vi "CreatePrivateEvents.vi"(8 "error in (no error)":errorcluster, 11 "Tool Data":refnum<class "Tool Data.lvclass">) -> (0 "error out":errorcluster, 3 "Tool Data out":refnum<class "Tool Data.lvclass">)   [LabVIEW 2019, in "Tool Data.lvclass"]
doc: "---------------------------------------------------------------\nJKI State Machine Objects™\nhttp://jki.net/state-machine-objects/\nCopyright (C) 2005-2015, JKI <info@jki.net>\nALL RIGHTS RESERVEDJKI State Machine Objects (SMO) 1.0.0.4\nJKI - JKI\nCopyright (c) 2015, JKI"
uses:
  Tool Data.lvclass
  Typedefs/PrivateEvents--Tool Data.Update Objects.ctl
  Settings/Setting Database/Typedefs/PublicEvents--Setting Database.PathsUpdated.ctl
  Settings/Path Settings/Path Settings.lvclass
  Settings/Setting Database/Typedefs/PublicEvents--Setting Database.RectanglesUpdated.ctl
  Settings/Rectangle Settings/Rectangle Settings.lvclass
  Settings/Setting Database/Typedefs/PublicEvents--Setting Database.FunnelsUpdated.ctl
  Settings/Funnel Settings/Funnel Settings.lvclass
  Settings/Setting Database/Typedefs/PublicEvents--Setting Database.DotsUpdated.ctl
  Settings/Dot Settings/Dot Settings.lvclass
  Parse/ParsePaths/Path.lvclass
  Parse/Rectangle/Rectangle.lvclass
  Parse/Image/SVGImage.lvclass
  Parse/Dot/Dot.lvclass
  Tool Data.lvclass/Tool Data.ctl
  <vilib>/JKI/JKI SMO/SMO/SMO.lvclass
  Settings/Setting Database/Setting Database.lvclass
panel:
  # "For instructions on how to use the JKI State Machine Objects, examples and video tutorials, visit:\nhttp://jki.net/state-machine-objects/\n\nJKI State Machine Objects™\nhttp://jki.net/state-machine-objects/\nCopyright (C) 2005-2015, JKI <info@jki.net>\nALL RIGHTS RESERVED"
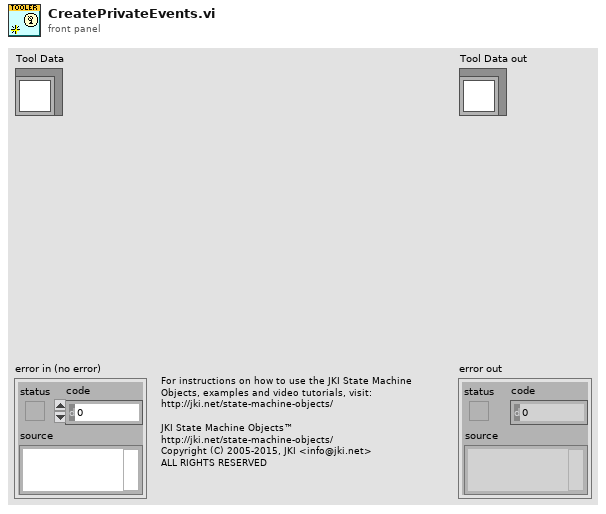
[diagram p1: front panel]
types:
  T1 = typedef "Tool Data.lvclass/PrivateEvents--Tool Data.Update Objects.ctl" = cluster{"Settings":cluster{"Paths":T2, "Rectangles":T3, "Funnels":T4, "Dots":T5}, "Data":cluster{"Paths":refnum<class "Path.lvclass">[], "Rectangles":refnum<class "Rectangle.lvclass">[], "SVGImage":refnum<class "SVGImage.lvclass">, "Dots":refnum<class "Dot.lvclass">[], "Funnels":refnum<class "Path.lvclass">[]}}
  T2 = typedef "Setting Database.lvclass/PublicEvents--Setting Database.PathsUpdated.ctl" = refnum<class "Path Settings.lvclass">[]
  T3 = typedef "Setting Database.lvclass/PublicEvents--Setting Database.RectanglesUpdated.ctl" = refnum<class "Rectangle Settings.lvclass">[]
  T4 = typedef "Setting Database.lvclass/PublicEvents--Setting Database.FunnelsUpdated.ctl" = refnum<class "Funnel Settings.lvclass">[]
  T5 = typedef "Setting Database.lvclass/PublicEvents--Setting Database.DotsUpdated.ctl" = refnum<class "Dot Settings.lvclass">[]
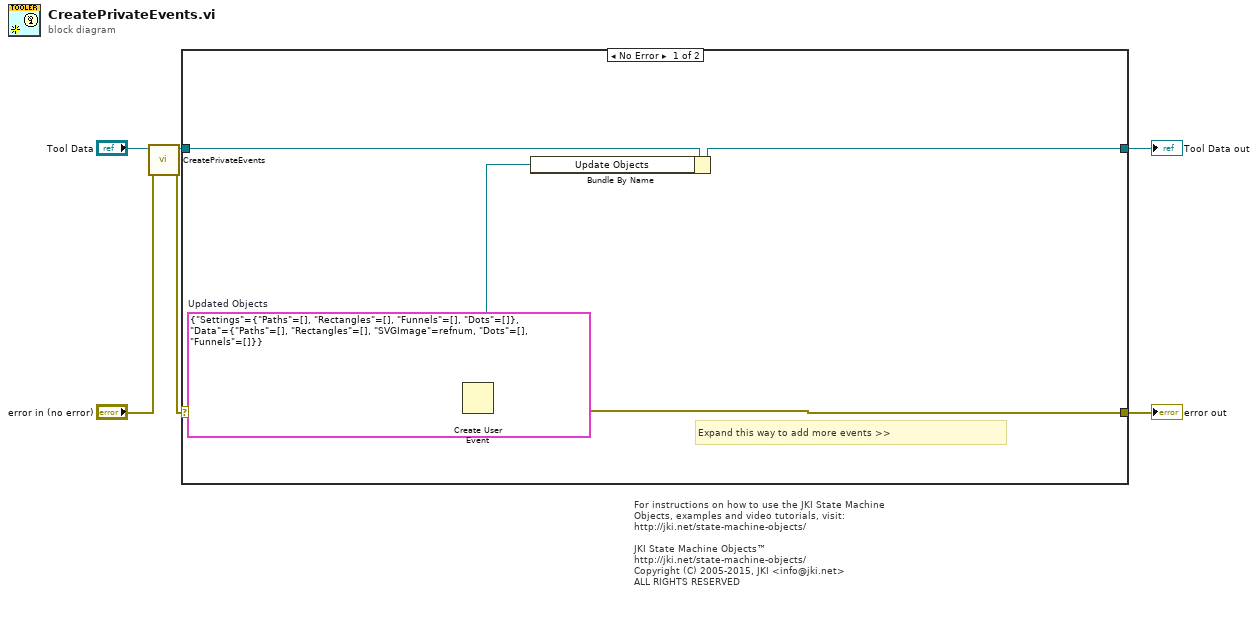
[diagram p0: block diagram]
diagram:
  # "For instructions on how to use the JKI State Machine Objects, examples and video tutorials, visit:\nhttp://jki.net/state-machine-objects/\n\nJKI State Machine Objects™\nhttp://jki.net/state-machine-objects/\nCopyright (C) 2005-2015, JKI <info@jki.net>\nALL RIGHTS RESERVED"
  n1 = call-parent "CreatePrivateEvents.vi"("error in (no error)"="error in (no error)", "SMO"="Tool Data") -> ("error out"=w1:errorcluster, "SMO out"=w3:refnum<class "Tool Data.lvclass">)  [unwired: 8 in]
  n2 = case shown="No Error" w1 {
    selector: w1 -> [w11 w14]
    tunnel: [w9 w14] -> w5
    tunnel: [w10 w13] -> w6
    tunnel: w3 -> [w12 w13]
    frame No Error {
      w8 = T1 {"Settings"={"Paths"=[], "Rectangles"=[], "Funnels"=[], "Dots"=[]}, "Data"={"Paths"=[], "Rectangles"=[], "SVGImage"=refnum, "Dots"=[], "Funnels"=[]}}  # Updated Objects
      # "Expand this way to add more events >>"
      n3 = Create User Event(user event datatype=w8, error in=w11) -> (user event=w7:refnum<user-event>, error out=w9:errorcluster)
      n4 = Bundle By Name(cluster=w12, "Update Objects"=w7) -> (w10:refnum<class "Tool Data.lvclass">)
    }
    frame Error {
    }
  }
  "error out" <- w5
  "Tool Data out" <- w6
